vi "AnalyzeEvent.vi"(6 "Max triggers?":bool, 9 "Channel - Current":u32, 10 "Channel - Previous":u32) -> (3 "Analyze?":bool)   [LabVIEW 2023]
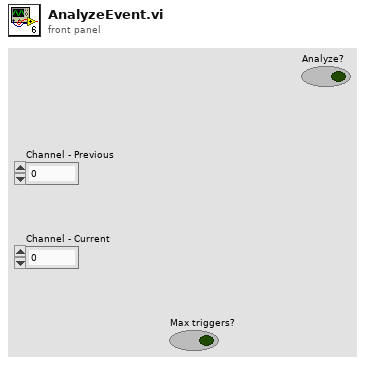
[diagram p1: front panel]
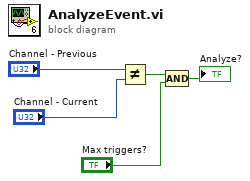
[diagram p0: block diagram]
diagram:
  n1 = Not Equal?(x="Channel - Previous", y="Channel - Current") -> (x != y?=w2:bool)
  n2 = Compound Arithmetic op=AND(w2, "Max triggers?") -> (→"Analyze?":bool)
